vi "Handle New Config.vi"(8 "error in (no error)":errorcluster, 10 "Request":refnum<class "Request.lvclass">, 11 "ConfigHTTPController in":refnum<class "ConfigHTTPController.lvclass">) -> (0 "error out":errorcluster, 3 "ConfigHTTPController out":refnum<class "ConfigHTTPController.lvclass">)   [LabVIEW 2020, in "Volatus.lvlib" / "ConfigHTTPController.lvclass"]
uses:
  ConfigHTTPController.lvclass
  ConfigHTTPController.lvclass/ConfigHTTPController.ctl
  lv-http-util/HTTP Utils/Request/Request.lvclass
  lv-http-util/HTTP Utils/FormField/FormField.lvclass
  MessageQ/MessageQ.lvclass
  New Config.ctl
  Volatus.lvlib
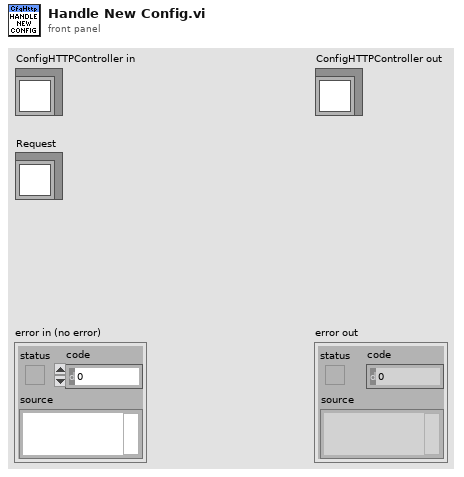
[diagram p1: front panel]
types:
  T1 = typedef "Volatus.lvlib/New Config.ctl" = cluster{"System":string, "Cluster":string, "Node":string, "Config":string}
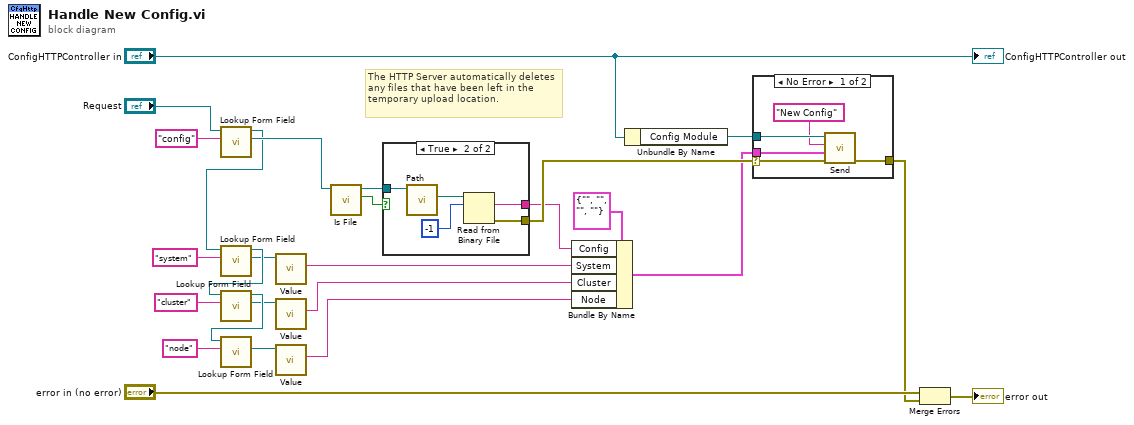
[diagram p0: block diagram]
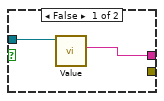
[diagram p3: hidden frame]
diagram:
  # "The HTTP Server automatically deletes any files that have been left in the temporary upload location."
  n1 = call "Lookup Form Field.vi"("Name"="config", "Request in"="Request") -> ("Field"=w23:refnum<class "FormField.lvclass">, "Request out"=w14:refnum<class "Request.lvclass">)  [unwired: 6 in, 2 out]
  n2 = call "Lookup Form Field.vi"("Name"="system", "Request in"=w14) -> ("Field"=w8:refnum<class "FormField.lvclass">, "Request out"=w13:refnum<class "Request.lvclass">)  [unwired: 6 in, 2 out]
  n3 = call "Lookup Form Field.vi"("Name"="cluster", "Request in"=w13) -> ("Field"=w7:refnum<class "FormField.lvclass">, "Request out"=w12:refnum<class "Request.lvclass">)  [unwired: 6 in, 2 out]
  n4 = call "Lookup Form Field.vi"("Name"="node", "Request in"=w12) -> ("Field"=w6:refnum<class "FormField.lvclass">)  [unwired: 6 in, 3 out]
  n5 = call "Value.vi"("FormField in"=w8) -> ("Value"=w5:string)  [unwired: 8 in, 2 out]
  n6 = call "Value.vi"("FormField in"=w7) -> ("Value"=w4:string)  [unwired: 8 in, 2 out]
  n7 = call "Value.vi"("FormField in"=w6) -> ("Value"=w3:string)  [unwired: 8 in, 2 out]
  n8 = call "Is File.vi"("FormField in"=w23) -> ("Is File?"=w22:bool, "FormField out"=w21:refnum<class "FormField.lvclass">)  [unwired: 8 in, 1 out]
  n9 = case shown="True" w22 {
    tunnel: [w28 w30] -> w9
    tunnel: w21 -> [w27 w33]
    tunnel: [_ w29] -> w20
    frame False {
      n10 = call "Value.vi"("FormField in"=w27) -> ("Value"=w28:string)  [unwired: 8 in, 2 out]
    }
    frame True {
      n11 = call "Path.vi"("FormField in"=w33) -> ("Path"=w32:path)  [unwired: 8 in, 2 out]
      n12 = Read from Binary File(10:-1 ("count (1)"), 11:w32) -> (0:w29:errorcluster, 2:w30:string)  [unwired: 4 in, 2 out]
    }
  }
  n13 = Bundle By Name(cluster=T1 {"System"="", "Cluster"="", "Node"="", "Config"=""} ("New Config"), "Config"=w9, "System"=w5, "Cluster"=w4, "Node"=w3) -> (w10:T1)
  n14 = Unbundle By Name("ConfigHTTPController in") -> ("Config Module"=w25:refnum<class "MessageQ.lvclass">)
  n15 = case shown="No Error" w20 {
    selector: w20 -> [w35 w39]
    tunnel: w25 -> [w38 _]
    tunnel: [w36 w39] -> w1
    tunnel: w10 -> [w34 _]
    frame No Error {
      n16 = call "Send.vi"("error in (no error)"=w35, "Data"=w34, "ID"="New Config", "MessageQ in"=w38) -> ("error out"=w36:errorcluster)  [unwired: 6 in, 1 out]
    }
    frame Error {
    }
  }
  n17 = Merge Errors("error in (no error)", w1) -> (→"error out":errorcluster)
  "ConfigHTTPController out" <- "ConfigHTTPController in"
